vi "Check If Parent Missile.vi"(9 "GB Components in":refnum<class "Game Board Component.lvclass">[](array[class]), 11 "Flying Saucer in":refnum<class "Flying Saucer.lvclass">) -> (2 "Not parent missile?":bool)   [LabVIEW 2021, in "Flying Saucer.lvclass"]
doc: "MIT Licence\nCopyright (c) 2024 David Grollier"
uses:
  Flying Saucer.lvclass
  Game Board Component.lvclass
  Missile/Missile.lvclass
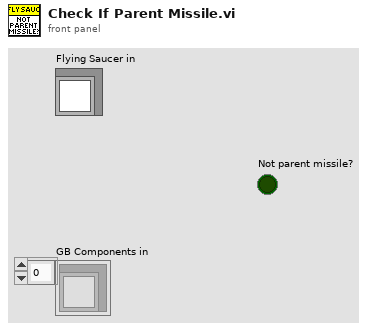
[diagram p1: front panel]
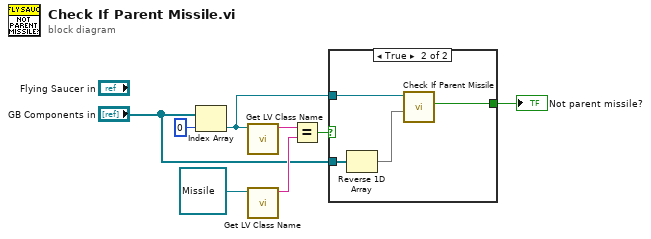
[diagram p0: block diagram]
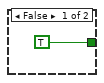
[diagram p2: hidden frame]
diagram:
  n1 = Index Array(array="GB Components in", index=0) -> (element=w4:refnum<class "Game Board Component.lvclass">)
  n2 = call <vilib>:"Get LV Class Name.vi"("object"=w4) -> ("class name"=w6:string)  [unwired: 9 in, 1 out]
  n3 = call <vilib>:"Get LV Class Name.vi"("object"=refnum<class "Missile.lvclass"> refnum ("Missile in")) -> ("class name"=w5:string)  [unwired: 9 in, 1 out]
  n4 = Equal?(x=w6, y=w5) -> (x = y?=w2:bool)
  n5 = case shown="True" w2 {
    tunnel: w4 -> [_ w13]
    tunnel: "GB Components in" -> [_ w12]
    tunnel: [TRUE ("Not parent missile?") w11] -> w1
    frame False {
    }
    frame True {
      n6 = Reverse 1D Array(array=w12) -> (reversed array=w10:refnum<class "Game Board Component.lvclass">[])
      n7 = call-dynamic "Check If Parent Missile.vi"("GB Components in"=w10, "Game Board Component in"=w13) -> ("Not parent missile?"=w11:bool)  [unwired: 9 in]
    }
  }
  "Not parent missile?" <- w1
